vi "Read Alarm - All.vi"(8 "error in (no error)":errorcluster, 11 "NT Base in":refnum<class "NT Base.lvclass">) -> (0 "error out":errorcluster, 2 "alarm":T1, 3 "NT Base out":refnum<class "NT Base.lvclass">)   [LabVIEW 2020, in "PV Access.lvlib" / "PV Data.lvlib" / "NT Base.lvclass"]
uses:
  NT Base.lvclass
  NT Base.lvclass/NT Base.ctl
  Alarm Severity.ctl
  PV Data.lvlib
  Alarm Status.ctl
  Alarm.ctl
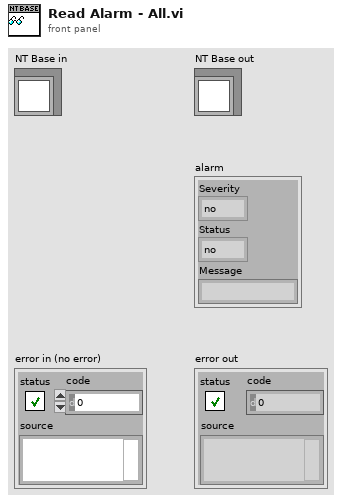
[diagram p1: front panel]
types:
  T1 = typedef "PV Access.lvlib/PV Data.lvlib/Alarm.ctl" = cluster{"Severity":T2, "Status":T3, "Message":string}
  T2 = typedef "PV Access.lvlib/PV Data.lvlib/Alarm Severity.ctl" = enum32{"no", "minor", "major", "record", "invalid", "undefined"}
  T3 = typedef "PV Access.lvlib/PV Data.lvlib/Alarm Status.ctl" = enum32{"no", "device", "driver", "record", "db", "conf", "undefined", "client"}
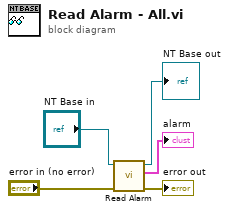
[diagram p0: block diagram]
diagram:
  n1 = call-dynamic "Read Alarm.vi"("error in"="error in (no error)", "Has Alarm in"="NT Base in") -> ("error out"=→"error out":errorcluster, "alarm"=→"alarm":T1, "Has Alarm out"=→"NT Base out":refnum<class "NT Base.lvclass">)  [unwired: 7 in]
